vi "TriggerMode_SaveImager.vi"() -> ()   [LabVIEW 2022 SP3]
panel:
  in  "Camera Control":bool
  in  "Trigger":bool
  out "Frame Rate":sgl
  in  "?":bool
  in  "Stop Grabbing":bool
  out "# of Iteration":i32
  in  "ActiveFlyCapControl":refnum<k7>(container)
  # "This is an simlple ActiveX example using methods provided by ActiveFlyCapConctrol to grab images from an PGR camera,  \ndisplay it on the screen and retrieve the frame rate at the same time. Also, it can toggle between free running mode and software\ntrigger mode. It is meant to let new users become farmiliar with the ActiveX control provided by the Flycapture SDK, so more compilcated blocks can be build upon."
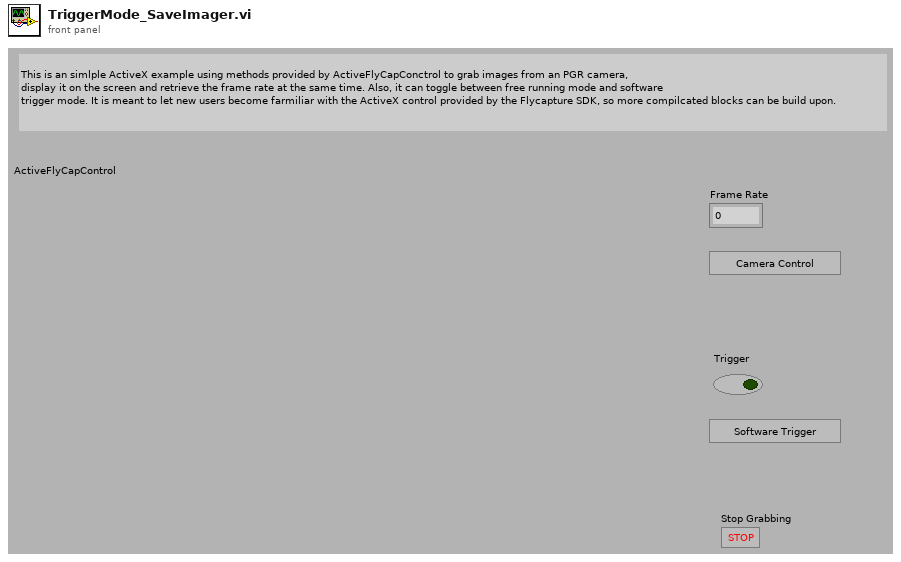
[diagram p1: front panel]
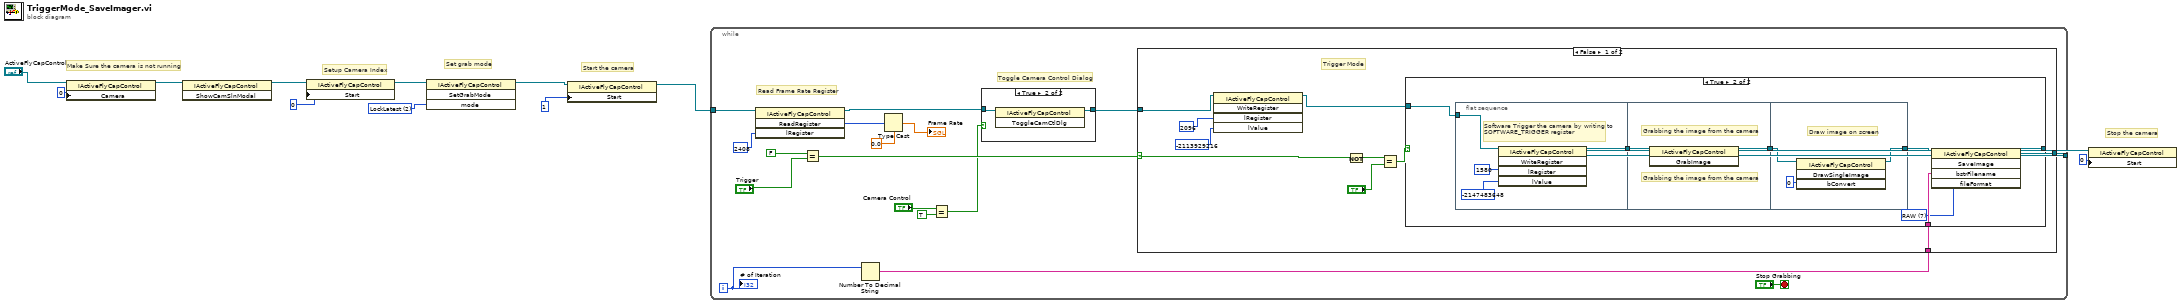
[diagram p0: block diagram]
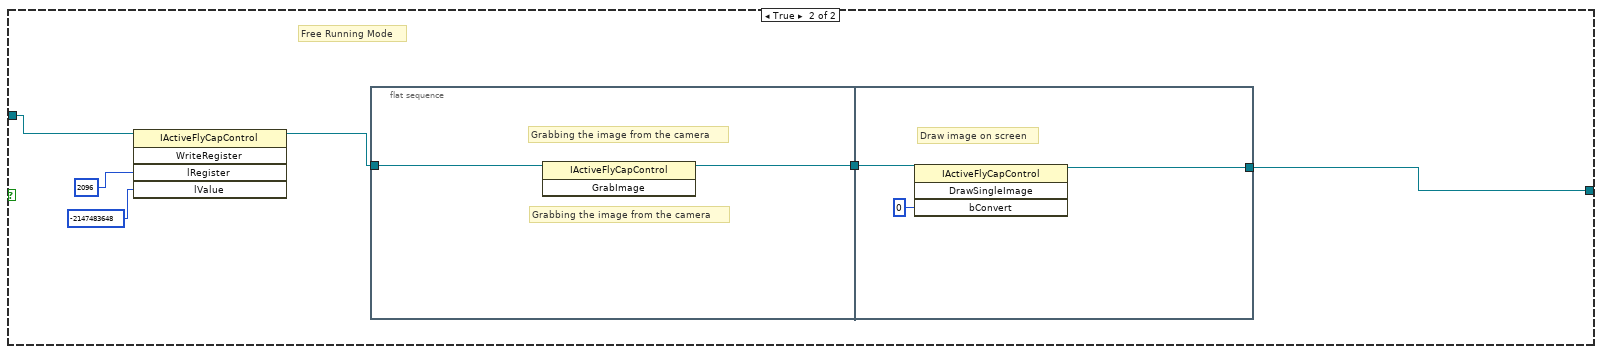
[diagram p4: hidden frame]
diagram:
  w12 = 2 items=["FreeRunning", "LockNext", "LockLatest"] ("mode")
  # "Start the camera"
  # "Stop the camera"
  # "Setup Camera Index"
  # "Set grab mode"
  # "Make Sure the camera is not running"
  n1 = property class="IActiveFlyCapControl"(reference="ActiveFlyCapControl", "Camera"=0 ("Start")) -> (reference out=w7:refnum<k7>)  [unwired: 1 in, 1 out]
  n2 = invoke class="IActiveFlyCapControl" method="ShowCamSlnModal"(reference=w7) -> (reference out=w6:refnum<k7>)  [unwired: 2 in, 2 out]
  n3 = property class="IActiveFlyCapControl"(reference=w6, "Start"=0 ("Camera")) -> (reference out=w8:refnum<k7>)  [unwired: 1 in, 1 out]
  n4 = invoke class="IActiveFlyCapControl" method="SetGrabMode"(reference=w8, "mode"=w12) -> (reference out=w1:refnum<k7>)  [unwired: 2 in, 3 out]
  n5 = property class="IActiveFlyCapControl"(reference=w1, "Start"=1) -> (reference out=w2:refnum<k7>)  [unwired: 1 in, 1 out]
  n6 = while {
    tunnel: w2 -> [w25]
    tunnel: [w28] -> w3
    i -> [w14]
    stop <- "Stop Grabbing" stop-if-true
    # "Read Frame Rate Register"
    # "Toggle Camera Control Dialog"
    n7 = invoke class="IActiveFlyCapControl" method="ReadRegister"(reference=w25, "lRegister"=2408) -> (reference out=w19:refnum<k7>, "ReadRegister"=w22:i32)  [unwired: 2 in, 2 out]
    n8 = Equal?(x=FALSE, y="Trigger") -> (x = y?=w26:bool)
    n9 = Number To Decimal String(number=w14) -> (decimal integer string=w13:string)  [unwired: 1 in]
    n10 = Type Cast(type=sgl 0.0 ("32-bit IEEE 754"), x=w22) -> (*(type *) &x=→"Frame Rate":sgl)
    n11 = Equal?(x="Camera Control", y=TRUE) -> (x = y?=w16:bool)
    n12 = case shown="True" w16 {
      tunnel: w19 -> [w30 w32]
      tunnel: [w30 w31] -> w15
      frame False {
      }
      frame True {
        n13 = invoke class="IActiveFlyCapControl" method="ToggleCamCtlDlg"(reference=w32) -> (reference out=w31:refnum<k7>)  [unwired: 2 in, 2 out]
      }
    }
    n14 = case shown="False" w26 {
      selector: w26 -> [w41 _]
      tunnel: [w42 w64] -> w28
      tunnel: w15 -> [w35 w61]
      tunnel: w13 -> [w33 _]
      frame False {
        # "Trigger Mode"
        n15 = invoke class="IActiveFlyCapControl" method="WriteRegister"(reference=w35, "lRegister"=2096, "lValue"=-2113929216 ("Register value in Hex 2")) -> (reference out=w34:refnum<k7>)  [unwired: 2 in, 4 out]
        n16 = Not(x=w41) -> (.not. x?=w40:bool)
        n17 = Equal?(x=w40, y="?") -> (x = y?=w38:bool)
        n18 = case shown="True" w38 {
          tunnel: [w43 w44] -> w42
          tunnel: w34 -> [w43 w48]
          tunnel: w33 -> [_ w47]
          frame False {
          }
          frame True {
            w46 = 7 items=["PGM", "PPM", "BMP", "JPEG", "JPEG2000", "TIFF", "PNG", "RAW"] ("fileFormat")
            n19 = flat-sequence {
              tunnel: [w52] -> w50
              tunnel: w48 -> [w51]
              tunnel: [w55] -> w49
              tunnel: w50 -> [w56]
              tunnel: w49 -> [w58]
              tunnel: [w57] -> w45
              frame #0 {
                # "Software Trigger the camera by writing to SOFTWARE_TRIGGER register"
                n20 = invoke class="IActiveFlyCapControl" method="WriteRegister"(reference=w51, "lRegister"=1580, "lValue"=-2147483648 ("Register value in Hex 2")) -> (reference out=w52:refnum<k7>)  [unwired: 2 in, 4 out]
              }
              frame #1 {
                # "Grabbing the image from the camera"
                # "Grabbing the image from the camera"
                n21 = invoke class="IActiveFlyCapControl" method="GrabImage"(reference=w56) -> (reference out=w55:refnum<k7>)  [unwired: 2 in, 2 out]
              }
              frame #2 {
                # "Draw image on screen"
                n22 = invoke class="IActiveFlyCapControl" method="DrawSingleImage"(reference=w58, "bConvert"=0) -> (reference out=w57:refnum<k7>)  [unwired: 2 in, 3 out]
              }
            }
            n23 = invoke class="IActiveFlyCapControl" method="SaveImage"(reference=w45, "bstrFilename"=w47, "fileFormat"=w46) -> (reference out=w44:refnum<k7>)  [unwired: 2 in, 4 out]
          }
        }
      }
      frame True {
        # "Free Running Mode"
        n24 = invoke class="IActiveFlyCapControl" method="WriteRegister"(reference=w61, "lRegister"=2096, "lValue"=-2147483648 ("Register value in Hex 2")) -> (reference out=w60:refnum<k7>)  [unwired: 2 in, 4 out]
        n25 = flat-sequence {
          tunnel: [w67] -> w65
          tunnel: w60 -> [w66]
          tunnel: w65 -> [w70]
          tunnel: [w69] -> w64
          frame #0 {
            # "Grabbing the image from the camera"
            # "Grabbing the image from the camera"
            n26 = invoke class="IActiveFlyCapControl" method="GrabImage"(reference=w66) -> (reference out=w67:refnum<k7>)  [unwired: 2 in, 2 out]
          }
          frame #1 {
            # "Draw image on screen"
            n27 = invoke class="IActiveFlyCapControl" method="DrawSingleImage"(reference=w70, "bConvert"=0) -> (reference out=w69:refnum<k7>)  [unwired: 2 in, 3 out]
          }
        }
      }
    }
    "# of Iteration" <- w14
  }
  n28 = property class="IActiveFlyCapControl"(reference=w3, "Start"=0) -> ()  [unwired: 1 in, 2 out]
